vi "LDA2_Safety.vi"(1 "Adam Loop Count":i32, 2 "Ch Names":string[](array[string]), 3 "Values":dbl[](array[numeric]) format="%.2f") -> (0 "Scan comment":string)   [LabVIEW 2021]
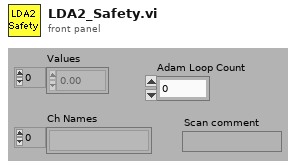
[diagram p1: front panel]
types:
  T1 = typedef "LVDateTimeRec.ctl" = cluster{"fractional second":dbl, "second":i32, "minute":i32, "hour":i32, "day of month":i32, "month":i32, "year":i32, "day of week":i32, "day of year":i32, "DST":i32}
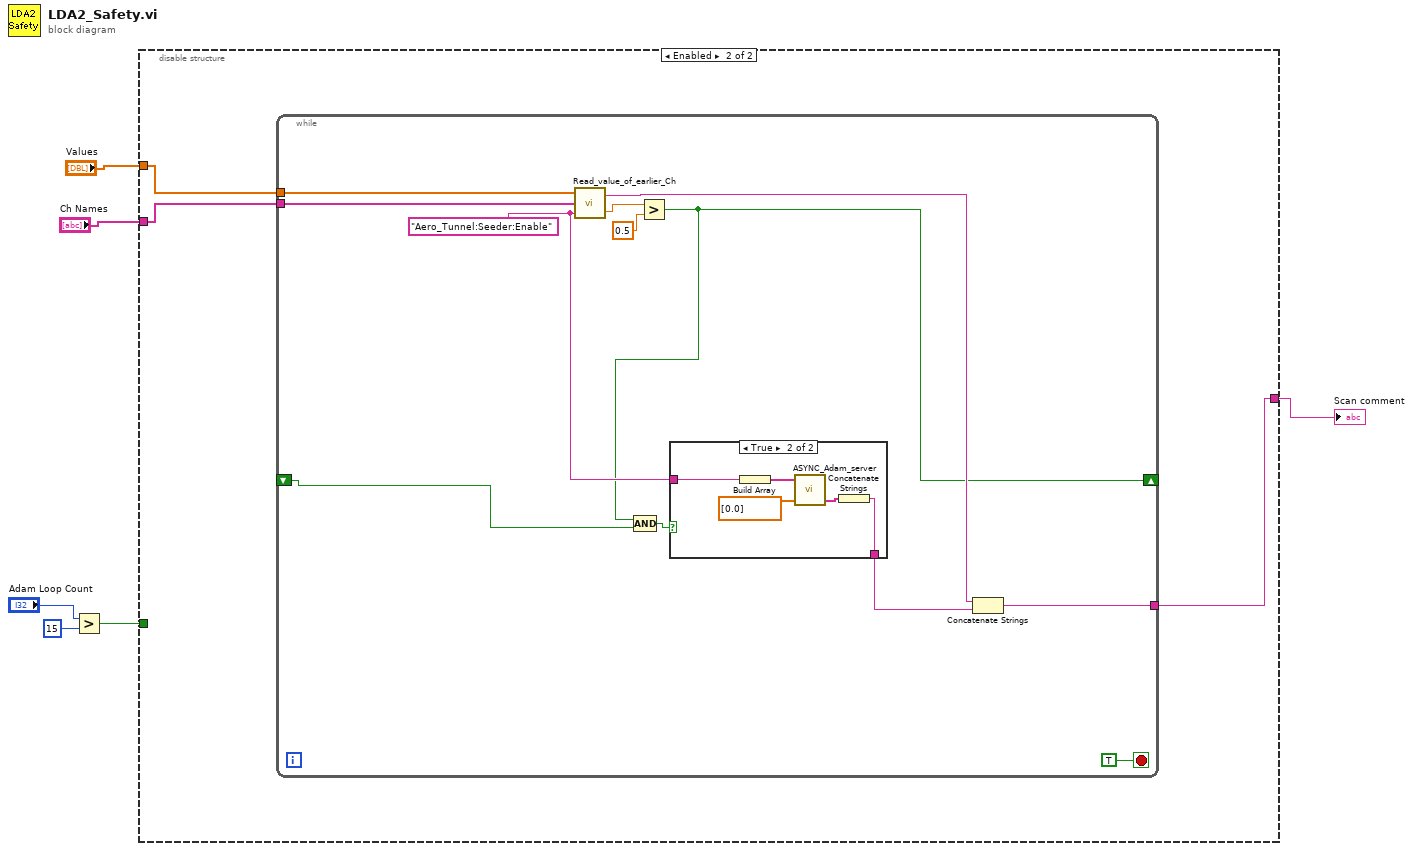
[diagram p0: block diagram]
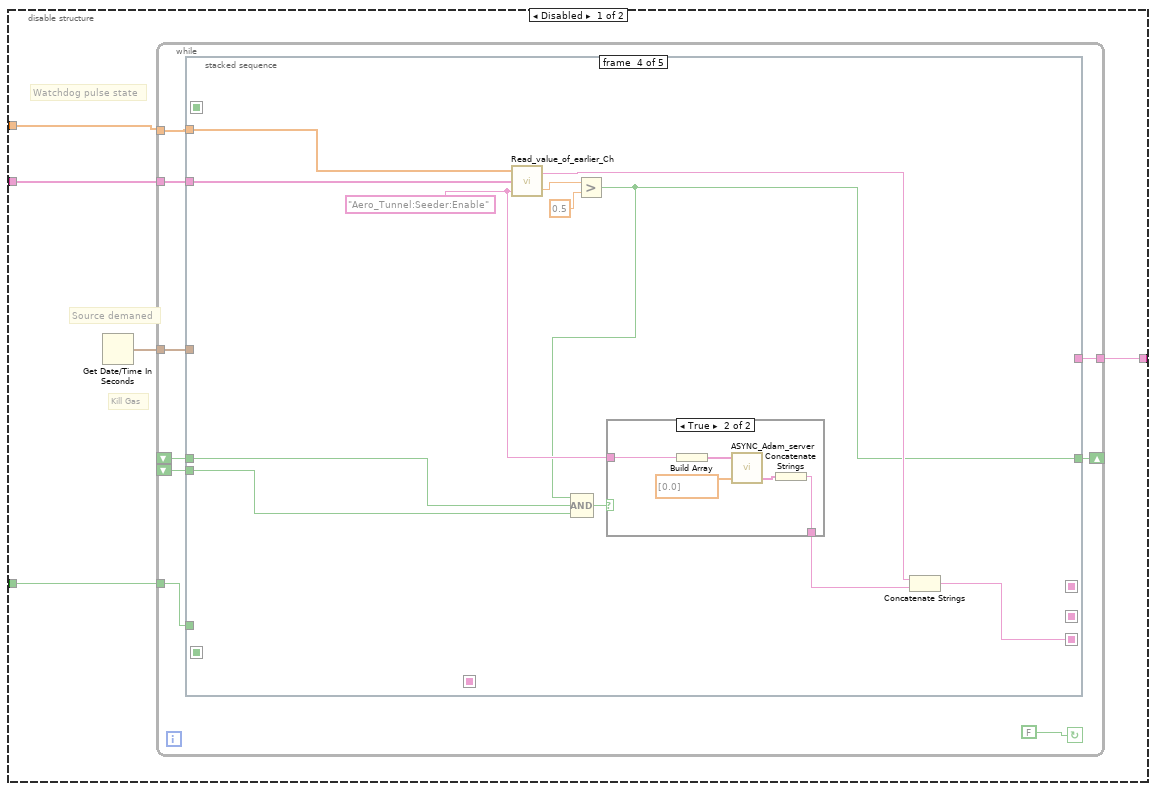
[diagram p2: hidden frame]
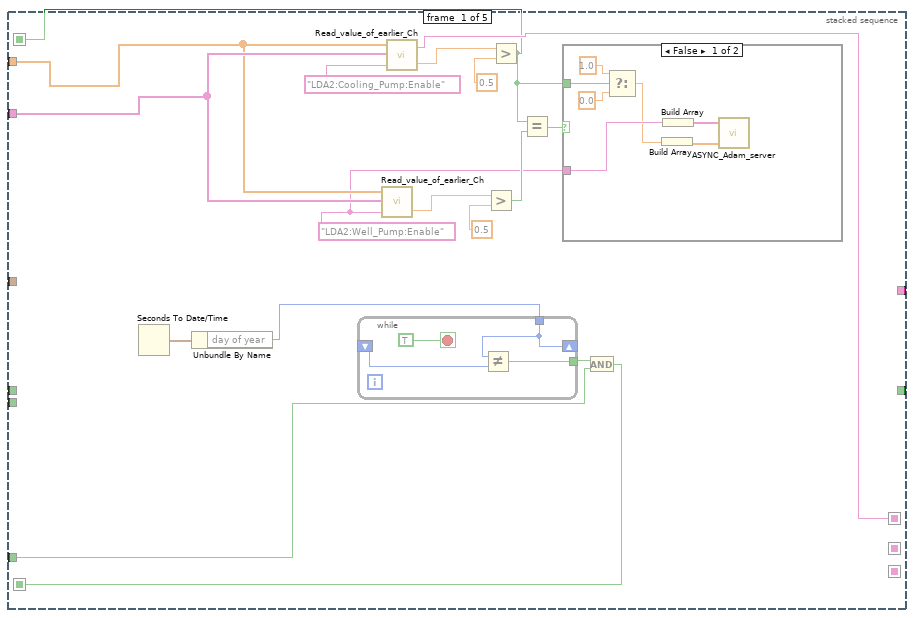
[diagram p3: hidden frame]
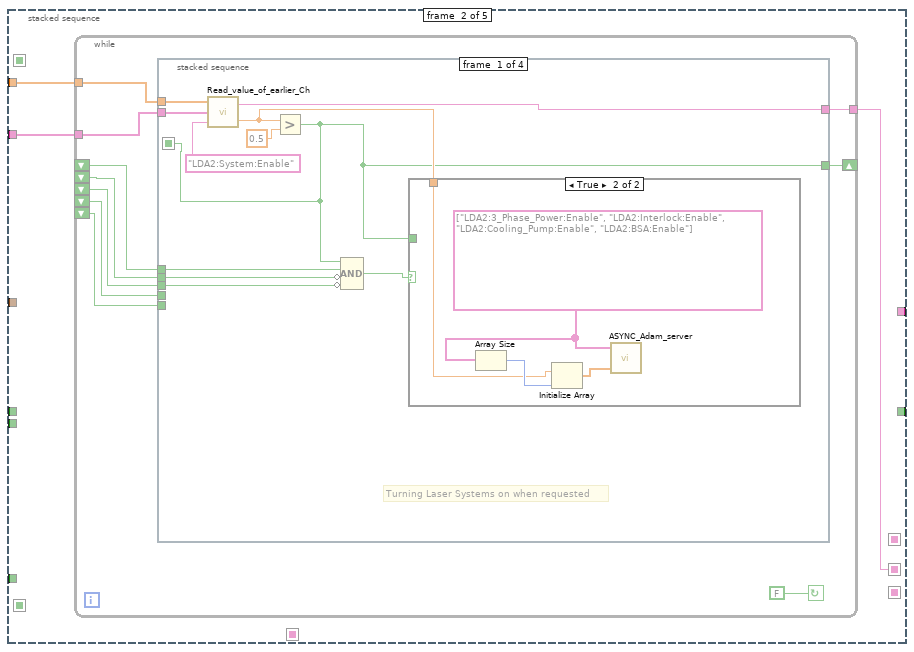
[diagram p5: hidden frame]
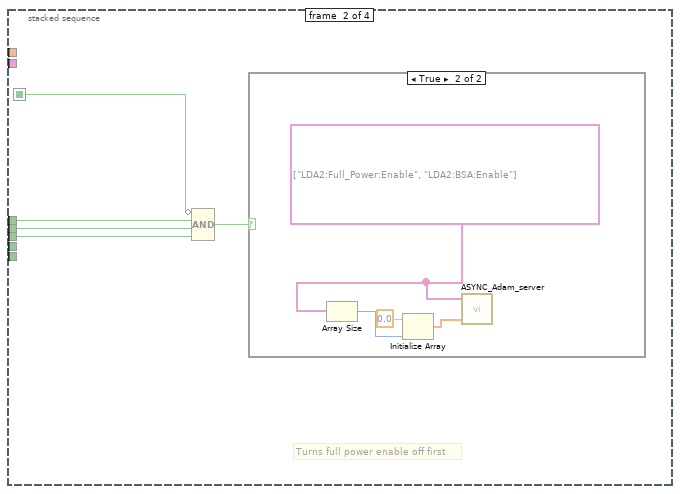
[diagram p7: hidden frame]
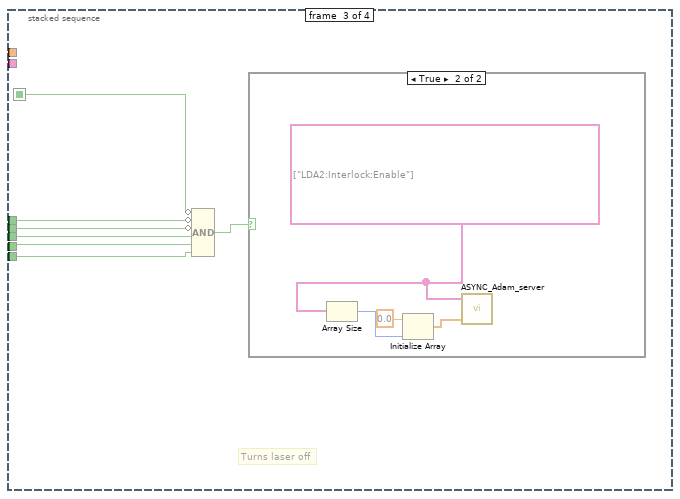
[diagram p9: hidden frame]
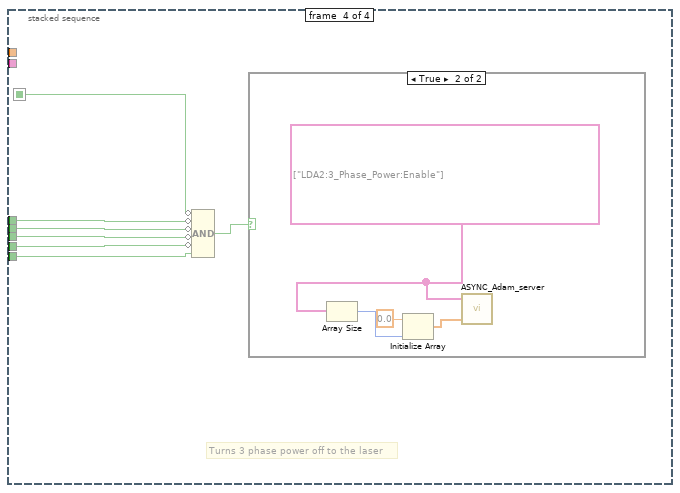
[diagram p11: hidden frame]
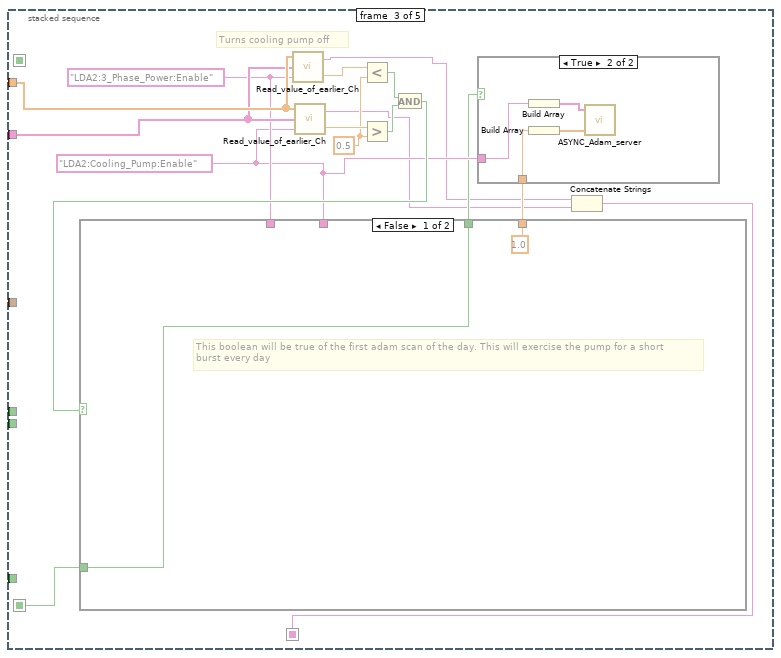
[diagram p13: hidden frame]
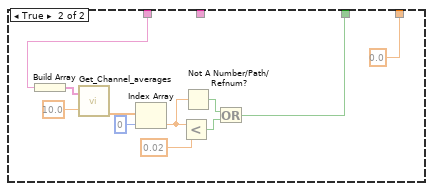
[diagram p15: hidden frame]
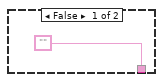
[diagram p16: hidden frame]
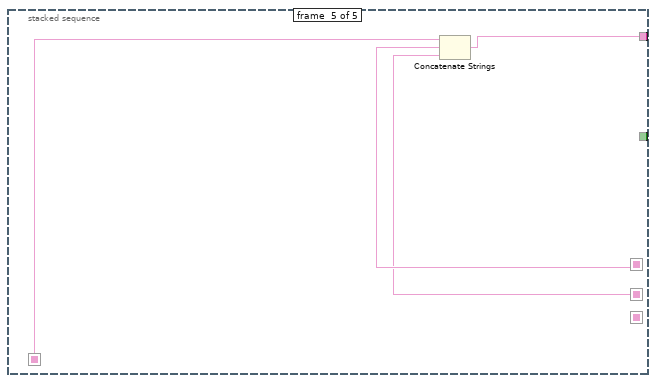
[diagram p17: hidden frame]
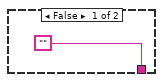
[diagram p18: hidden frame]
diagram:
  n1 = Greater?(x="Adam Loop Count", y=15) -> (0:w1:bool)
  n2 = disable-structure shown="Enabled" {
    disable-tunnel: [w10 w163] -> w6
    disable-tunnel: "Values" -> [w9 w165]
    disable-tunnel: "Ch Names" -> [w8 w164]
    disable-tunnel: w1 -> [w7 _]
    frame Disabled {
      # "Source demaned"
      # "Watchdog pulse state"
      # "Kill Gas"
      n3 = Get Date/Time In Seconds() -> (seconds since 1Jan1904=w11:timestamp)
      n4 = while {
        tunnel: w8 -> [w20]
        tunnel: w9 -> [w19]
        tunnel: w11 -> [w17]
        shift-right: [w16] -> _
        shift-left: _ -> [w15]
        shift-left: _ -> [w14]
        tunnel: [w13] -> w10
        tunnel: w7 -> [w12]
        stop <- FALSE continue-if-true
        n5 = stacked-sequence {
          seq-local: [w30 _ _ _ _] -> [_ _ w111 _ _]
          seq-local: [w21 _ _ _ _] -> [_ _ _ _ _]
          seq-local: [w34 _ _ _ _] -> [_ _ _ _ w162]
          seq-local: [_ w49 _ _ _] -> [_ _ _ _ w161]
          seq-local: [_ _ w108 _ _] -> [_ _ _ _ w160]
          seq-local: [_ _ _ w145 _] -> [_ _ _ _ _]
          tunnel: w20 -> [w26 w50 w121 w149 _]
          tunnel: w19 -> [w25 w51 w122 w150 _]
          tunnel: w12 -> [w29 _ _ _ _]
          tunnel: w17 -> [_ _ _ _ _]
          tunnel: [_ _ _ w144 _] -> w16
          tunnel: w15 -> [_ _ _ w143 _]
          tunnel: w14 -> [_ _ _ w142 _]
          tunnel: [_ _ _ _ w159] -> w13
          frame #0 {
            w22 = "LDA2:Well_Pump:Enable" ("Desired Ch to Read")
            n6 = Seconds To Date/Time() -> (date time rec=w33:T1)  [unwired: 2 in]
            n7 = Unbundle By Name(w33) -> ("day of year"=w32:i32)
            n8 = while {
              shift-right: [w48] -> _
              shift-left: _ -> [w47]
              tunnel: w32 -> [w48]
              tunnel: [w46] -> w31
              stop <- TRUE stop-if-true
              n9 = Not Equal?(x=w48, y=w47) -> (x != y?=w46:bool)
            }
            n10 = call "Read_value_of_earlier_Ch.vi"("Desired Ch to Read"=w22, "Ch names"=w26, "Present scan array"=w25) -> ("Value"=w27:dbl)  [unwired: 1 in, 1 out]
            n11 = call "Read_value_of_earlier_Ch.vi"("Desired Ch to Read"="LDA2:Cooling_Pump:Enable", "Ch names"=w26, "Present scan array"=w25) -> ("Value"=w36:dbl, "Scan comment"=w34:string)  [unwired: 1 in]
            n12 = Greater?(x=w27, y=0.5) -> (0:w24:bool)
            n13 = Greater?(x=w36, y=0.5) -> (0:w21:bool)
            n14 = Equal?(x=w21, y=w24) -> (x = y?=w23:bool)
            n15 = case shown="False" w23 {
              tunnel: w22 -> [w43 _]
              tunnel: w21 -> [w42 _]
              frame False {
                n16 = Select(t=1.0, s=w42, f=0.0) -> (s? t:f=w39:dbl)
                n17 = Build Array(w39) -> (w38:dbl[])
                n18 = Build Array(w43) -> (w44:string[])
                n19 = call "ASYNC_Adam_server.vi"("Values"=w38, "Channel Names"=w44) -> ()  [unwired: 1 in, 3 out]
              }
              frame True {
              }
            }
            n20 = And(x=w31, y=w29) -> (x .and. y?=w30:bool)
          }
          frame #1 {
            n21 = while {
              tunnel: w51 -> [w61]
              tunnel: w50 -> [w60]
              shift-right: [w55] -> _
              shift-left: _ -> [w58]
              shift-left: _ -> [w57]
              shift-left: _ -> [w56]
              tunnel: [w54] -> w49
              shift-left: _ -> [w53]
              shift-left: _ -> [w52]
              stop <- FALSE continue-if-true
              n22 = stacked-sequence {
                seq-local: [w63 _ _ _] -> [_ w78 w89 w100]
                tunnel: w61 -> [w72 _ _ _]
                tunnel: w60 -> [w71 _ _ _]
                tunnel: w58 -> [w67 w81 w92 w103]
                tunnel: w57 -> [w66 w80 w91 w102]
                tunnel: w56 -> [w65 w79 w90 w101]
                tunnel: [w63 _ _ _] -> w55
                tunnel: [w64 _ _ _] -> w54
                tunnel: w53 -> [_ _ w87 w98]
                tunnel: w52 -> [_ _ w86 w97]
                frame #0 {
                  # "Turning Laser Systems on when requested"
                  n23 = call "Read_value_of_earlier_Ch.vi"("Desired Ch to Read"="LDA2:System:Enable", "Ch names"=w71, "Present scan array"=w72) -> ("Value"=w68:dbl, "Scan comment"=w64:string)  [unwired: 1 in]
                  n24 = Greater?(x=w68, y=0.5) -> (0:w63:bool)
                  n25 = Compound Arithmetic op=AND(w63, w67, invert w66, invert w65) -> (w62:bool)
                  n26 = case shown="True" w62 {
                    tunnel: w68 -> [_ w73]
                    tunnel: w63 -> [_ _]
                    frame False {
                    }
                    frame True {
                      w76 = string[] ["LDA2:3_Phase_Power:Enable", "LDA2:Interlock:Enable", "LDA2:Cooling_Pump:Enable", "LDA2:BSA:Enable"] ("Channel Names")
                      n27 = Array Size(array=w76) -> (size(s)=w74:i32)
                      n28 = Initialize Array(w73, w74) -> (w75:dbl[])
                      n29 = call "ASYNC_Adam_server.vi"("Values"=w75, "Channel Names"=w76) -> ()  [unwired: 1 in, 3 out]
                    }
                  }
                }
                frame #1 {
                  # "Turns full power enable off first"
                  n30 = Compound Arithmetic op=AND(invert w78, w81, w80, w79) -> (w77:bool)
                  n31 = case shown="True" w77 {
                    frame False {
                    }
                    frame True {
                      w82 = string[] ["LDA2:Full_Power:Enable", "LDA2:BSA:Enable"] ("Channel Names")
                      n32 = Array Size(array=w82) -> (size(s)=w84:i32)
                      n33 = Initialize Array(0.0, w84) -> (w85:dbl[])
                      n34 = call "ASYNC_Adam_server.vi"("Values"=w85, "Channel Names"=w82) -> ()  [unwired: 1 in, 3 out]
                    }
                  }
                }
                frame #2 {
                  # "Turns laser off"
                  n35 = Compound Arithmetic op=AND(invert w89, invert w92, invert w91, w90, w87, w86) -> (w88:bool)
                  n36 = case shown="True" w88 {
                    frame False {
                    }
                    frame True {
                      w93 = string[] ["LDA2:Interlock:Enable"] ("Channel Names")
                      n37 = Array Size(array=w93) -> (size(s)=w95:i32)
                      n38 = Initialize Array(0.0, w95) -> (w96:dbl[])
                      n39 = call "ASYNC_Adam_server.vi"("Values"=w96, "Channel Names"=w93) -> ()  [unwired: 1 in, 3 out]
                    }
                  }
                }
                frame #3 {
                  # "Turns 3 phase power off to the laser"
                  n40 = Compound Arithmetic op=AND(invert w100, invert w103, invert w102, invert w101, invert w98, w97) -> (w99:bool)
                  n41 = case shown="True" w99 {
                    frame False {
                    }
                    frame True {
                      w104 = string[] ["LDA2:3_Phase_Power:Enable"] ("Channel Names")
                      n42 = Array Size(array=w104) -> (size(s)=w106:i32)
                      n43 = Initialize Array(0.0, w106) -> (w107:dbl[])
                      n44 = call "ASYNC_Adam_server.vi"("Values"=w107, "Channel Names"=w104) -> ()  [unwired: 1 in, 3 out]
                    }
                  }
                }
              }
            }
          }
          frame #2 {
            w115 = "LDA2:3_Phase_Power:Enable" ("Desired Ch to Read")
            w120 = 0.5 ("y")
            w114 = "LDA2:Cooling_Pump:Enable" ("Desired Ch to Read")
            # "Turns cooling pump off"
            n45 = call "Read_value_of_earlier_Ch.vi"("Desired Ch to Read"=w115, "Ch names"=w121, "Present scan array"=w122) -> ("Value"=w119:dbl, "Scan comment"=w110:string)  [unwired: 1 in]
            n46 = call "Read_value_of_earlier_Ch.vi"("Desired Ch to Read"=w114, "Ch names"=w121, "Present scan array"=w122) -> ("Value"=w123:dbl, "Scan comment"=w109:string)  [unwired: 1 in]
            n47 = Less?(x=w119, y=w120) -> (x < y?=w118:bool)
            n48 = Greater?(x=w123, y=w120) -> (0:w117:bool)
            n49 = And(x=w118, y=w117) -> (x .and. y?=w116:bool)
            n50 = case shown="False" w116 {
              tunnel: w115 -> [_ w135]
              tunnel: w114 -> [_ _]
              tunnel: [w128 w130] -> w113
              tunnel: [1.0 ("element") 0.0 ("element")] -> w112
              tunnel: w111 -> [w128 _]
              frame False {
                # "This boolean will be true of the first adam scan of the day. This will exercise the pump for a short\nburst every day"
              }
              frame True {
                n51 = Build Array(w135) -> (w139:string[])
                n52 = call "Get_Channel_averages.vi"("Desired Ch Names"=w139, "Averaging time (mins)"=10.0) -> ("number"=w138:dbl[])  [unwired: 1 in, 2 out]
                n53 = Index Array(array=w138, index=0) -> (element=w133:dbl)
                n54 = Less?(x=w133, y=0.02) -> (x < y?=w132:bool)
                n55 = Not A Number/Path/Refnum?(number/path/refnum=w133) -> (NaN/Path/Refnum?=w131:bool)
                n56 = Or(x=w131, y=w132) -> (x .or. y?=w130:bool)
              }
            }
            n57 = case shown="True" w113 {
              tunnel: w114 -> [_ w125]
              tunnel: w112 -> [_ w124]
              frame False {
              }
              frame True {
                n58 = Build Array(w125) -> (w126:string[])
                n59 = Build Array(w124) -> (w127:dbl[])
                n60 = call "ASYNC_Adam_server.vi"("Values"=w127, "Channel Names"=w126) -> ()  [unwired: 1 in, 3 out]
              }
            }
            n61 = Concatenate Strings(w110, w109) -> (w108:string)
          }
          frame #3 {
            w148 = "Aero_Tunnel:Seeder:Enable" ("Desired Ch to Read")
            n62 = call "Read_value_of_earlier_Ch.vi"("Desired Ch to Read"=w148, "Ch names"=w149, "Present scan array"=w150) -> ("Value"=w151:dbl, "Scan comment"=w147:string)  [unwired: 1 in]
            n63 = Greater?(x=w151, y=0.5) -> (0:w144:bool)
            n64 = Compound Arithmetic op=AND(w144, w143, w142) -> (w141:bool)
            n65 = case shown="True" w141 {
              tunnel: w148 -> [_ w158]
              tunnel: ["" w154] -> w146
              frame False {
              }
              frame True {
                n66 = Build Array(w158) -> (w157:string[])
                n67 = call "ASYNC_Adam_server.vi"("Values"=dbl[] [0.0], "Channel Names"=w157) -> ("Scan Comments"=w155:string[])  [unwired: 1 in, 2 out]
                n68 = Concatenate Strings(w155) -> (w154:string)
              }
            }
            n69 = Concatenate Strings(w147, w146) -> (w145:string)
          }
          frame #4 {
            n70 = Concatenate Strings(w160, w162, w161) -> (w159:string)
          }
        }
      }
    }
    frame Enabled {
      n71 = while {
        tunnel: w165 -> [w171]
        tunnel: w164 -> [w170]
        shift-right: [w169] -> _
        shift-left: _ -> [w168]
        tunnel: [w167] -> w163
        stop <- TRUE stop-if-true
        w175 = "Aero_Tunnel:Seeder:Enable" ("Desired Ch to Read")
        n72 = call "Read_value_of_earlier_Ch.vi"("Desired Ch to Read"=w175, "Ch names"=w170, "Present scan array"=w171) -> ("Value"=w176:dbl, "Scan comment"=w174:string)  [unwired: 1 in]
        n73 = Greater?(x=w176, y=0.5) -> (0:w169:bool)
        n74 = Compound Arithmetic op=AND(w169, w168) -> (w172:bool)
        n75 = case shown="True" w172 {
          tunnel: w175 -> [_ w183]
          tunnel: ["" w179] -> w173
          frame False {
          }
          frame True {
            n76 = Build Array(w183) -> (w182:string[])
            n77 = call "ASYNC_Adam_server.vi"("Values"=dbl[] [0.0], "Channel Names"=w182) -> ("Scan Comments"=w180:string[])  [unwired: 1 in, 2 out]
            n78 = Concatenate Strings(w180) -> (w179:string)
          }
        }
        n79 = Concatenate Strings(w174, w173) -> (w167:string)
      }
    }
  }
  "Scan comment" <- w6
